vi "Calculate and send speed.vi"(8 "error in (no error)":errorcluster, 11 "Autofocus in":refnum<class "Autofocus.lvclass">) -> (0 "error out":errorcluster, 3 "Autofocus out":refnum<class "Autofocus.lvclass">)   [LabVIEW 2012, in "Autofocus.lvclass"]
uses:
  Autofocus.lvclass
  <vilib>/Distrio/Murmex/Murmex/update_cluster.ctl
  Autofocus.lvclass/Autofocus.ctl
  <vilib>/Distrio/Murmex/Murmex/Murmex.lvclass
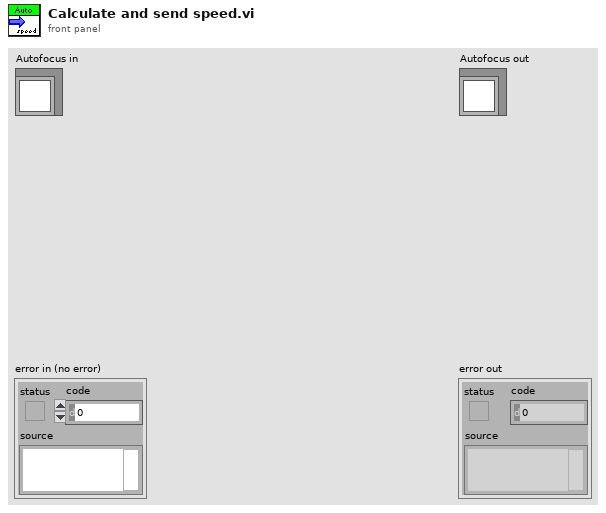
[diagram p1: front panel]
types:
  T1 = typedef "Murmex.lvlib/Murmex.lvclass/update_cluster.ctl" = cluster{"target ID":string, "key chains":string[], "values":variant[]}
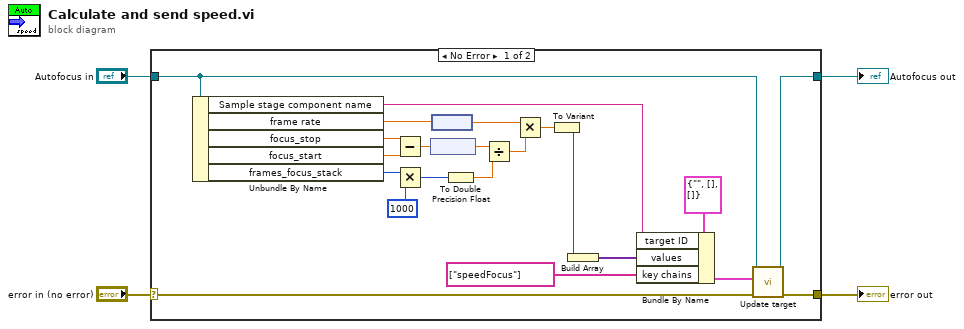
[diagram p0: block diagram]
diagram:
  n1 = case shown="No Error" "error in (no error)" {
    selector: "error in (no error)" -> [w13 w28]
    tunnel: [w12 w28] -> w3
    tunnel: [w10 w27] -> w1
    tunnel: "Autofocus in" -> [w11 w27]
    frame No Error {
      n2 = Unbundle By Name(w11) -> ("Sample stage component name"=w9:string, "frame rate"=w18:dbl[unit], "focus_stop"=w26:dbl[unit], "focus_start"=w25:dbl[unit], "frames_focus_stack"=w22:u16)
      n3 = Subtract(x=w26, y=w25) -> (x-y=w24:dbl[unit])
      n4 = Multiply(x=w22, y=u16 1000) -> (x*y=w20:u16)
      n5 = node(w24) -> (w23:dbl)
      n6 = node(w18) -> (w16:dbl)
      n7 = To Double Precision Float(number=w20) -> (double precision float=w19:dbl)
      n8 = Divide(x=w23, y=w19) -> (x/y=w17:dbl)
      n9 = Multiply(x=w16, y=w17) -> (x*y=w8:dbl)
      n10 = To Variant(anything=w8) -> (Variant=w7:variant)
      n11 = Build Array(w7) -> (w6:variant[])
      n12 = Bundle By Name(cluster=T1 {"target ID"="", "key chains"=[], "values"=[]} ("update cluster"), "target ID"=w9, "values"=w6, "key chains"=string[] ["speedFocus"]) -> (w15:T1)
      n13 = call <vilib>:"Update target.vi"("error in (no error)"=w13, "update cluster"=w15, "MurmexBase in"=w11) -> ("error out"=w12:errorcluster, "MurmexBase out"=w10:refnum<class "Autofocus.lvclass">)  [unwired: 7 in]
    }
    frame Error {
    }
  }
  "error out" <- w3
  "Autofocus out" <- w1
